vi "生成CODMn data (子VI).vi"() -> (3 "data":T1)   [LabVIEW 2016, in "斯坦道CODMn.lvlib"]
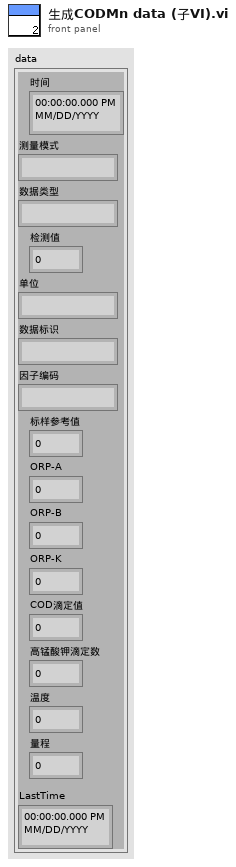
[diagram p1: front panel]
types:
  T1 = cluster{"时间":timestamp, "测量模式":string, "数据类型":string, "检测值":sgl, "单位":string, "数据标识":string, "因子编码":string, "标样参考值":sgl, "ORP-A":sgl, "ORP-B":sgl, "ORP-K":sgl, "COD滴定值":sgl, "高锰酸钾滴定数":sgl, "温度":sgl, "量程":sgl, "LastTime":timestamp}
  T2 = cluster{"运行模式":enum16{"维护模式", "常规模式", "应急模式", "质控模式"}}
  T3 = cluster{"测量量程":dbl, "测量精度":dbl, "测量间隔":dbl, "消解温度":dbl, "消解时长":dbl, "空白校准时间":timestamp, "曲线截距":dbl, "曲线斜率":dbl, "测量检出限":dbl, "测量信号值":dbl, "线性相关系数":dbl, "二次多项式系数":dbl, "标样校准时间":timestamp, "单位":u16}
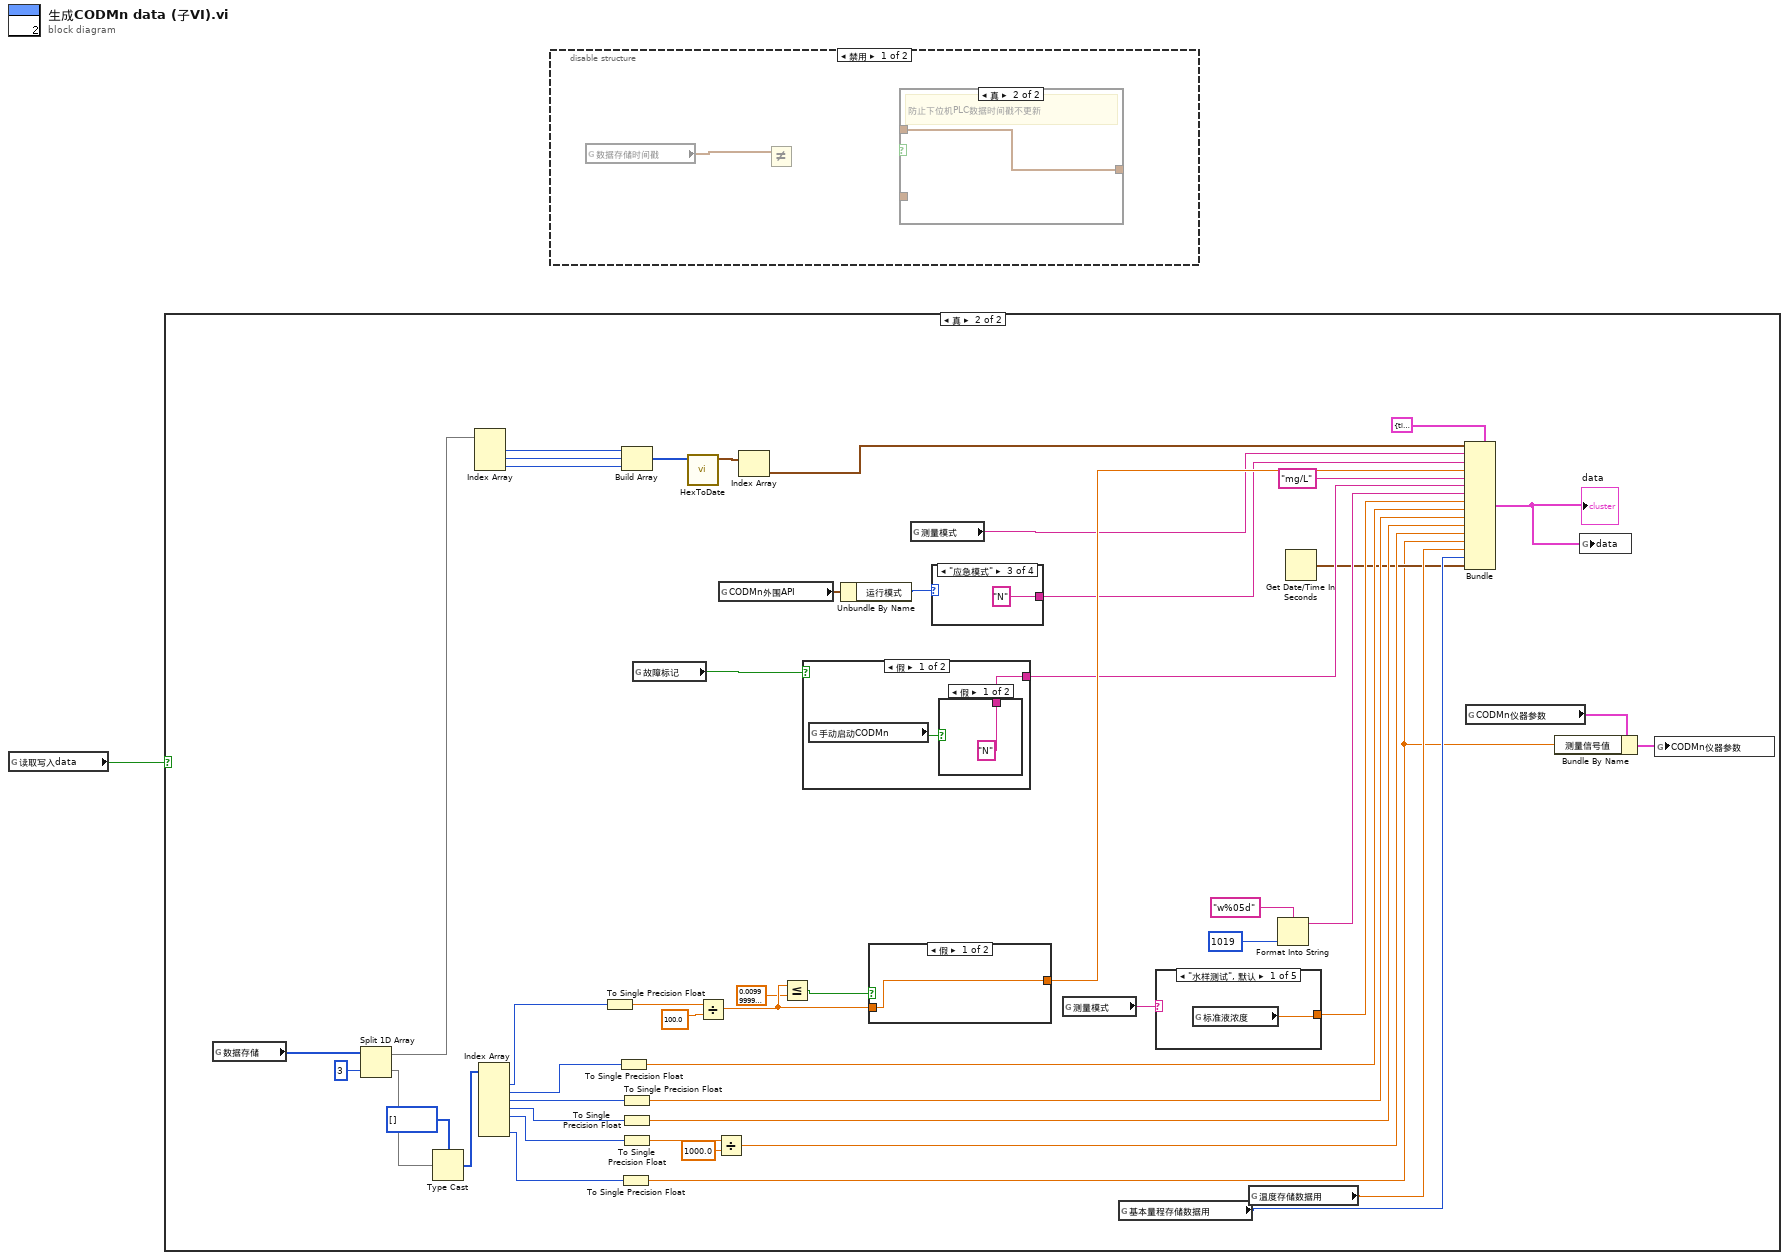
[diagram p0: block diagram]
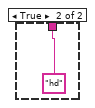
[diagram p5: hidden frame]
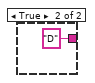
[diagram p6: hidden frame]
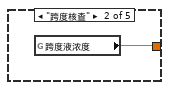
[diagram p7: hidden frame]
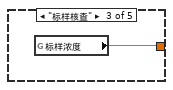
[diagram p8: hidden frame]
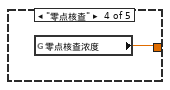
[diagram p9: hidden frame]
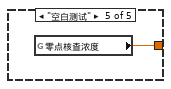
[diagram p10: hidden frame]
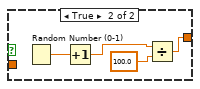
[diagram p11: hidden frame]
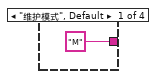
[diagram p12: hidden frame]
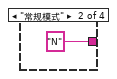
[diagram p13: hidden frame]
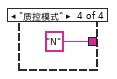
[diagram p14: hidden frame]
diagram:
  n1 = global read "COD内部交互全局.vi" "读取写入data"() -> (w1:bool)
  n2 = case shown="真" w1 {
    frame False {
    }
    frame True {
      n3 = global read "COD内部交互全局.vi" "数据存储"() -> (w9:u16[])
      n4 = Split 1D Array(array=w9, index=3 ("索引")) -> (first subarray=w15:u16[], second subarray=w8:u16[])
      n5 = Type Cast(type=i16[] [], x=w8) -> (*(type *) &x=w7:i16[])
      n6 = Index Array(array=w15) -> (element #1=w17:u16, element #2=w18:u16, element #3=w19:u16)  [unwired: 3 in]
      n7 = Index Array(array=w7) -> (element #1=w42:i16, element #2=w21:i16, element #3=w22:i16, element #4=w23:i16, element #5=w24:i16, element #7=w49:i16)  [unwired: 7 in, 1 out]
      n8 = To Single Precision Float(number=w42) -> (single precision float=w40:sgl)
      n9 = To Single Precision Float(number=w21) -> (single precision float=w33:sgl)
      n10 = To Single Precision Float(number=w49) -> (single precision float=w4:sgl)
      n11 = Build Array(w17, w18, w19) -> (w20:u16[])
      n12 = To Single Precision Float(number=w22) -> (single precision float=w32:sgl)
      n13 = To Single Precision Float(number=w23) -> (single precision float=w31:sgl)
      n14 = To Single Precision Float(number=w24) -> (single precision float=w27:sgl)
      n15 = global read "COD内部交互全局.vi" "故障标记"() -> (w51:bool)
      n16 = call "HexToDate.vi"("数组"=w20) -> ("DATE"=w16:timestamp[])  [unwired: 10 in]
      n17 = Divide(x=w40, y=sgl 100.0) -> (x/y=w41:sgl)
      n18 = Divide(x=w27, y=sgl 1000.0) -> (x/y=w30:sgl)
      n19 = global read "CODMN外部API.vi" "CODMn外围API"() -> (w45:T2)
      n20 = Index Array(array=w16) -> (element=w3:timestamp)  [unwired: 1 in]
      n21 = Less Or Equal?(x=w41, y=sgl 0.01) -> (x <= y?=w39:bool)
      n22 = case shown="假" w51 {
        tunnel: [w53 "D" ("数据标识")] -> w35
        frame False {
          n23 = global read "CODMN外部API.vi" "手动启动CODMn"() -> (w52:bool)
          n24 = case shown="假" w52 {
            tunnel: ["N" ("数据标识") "hd" ("数据标识")] -> w53
            frame False {
            }
            frame True {
            }
          }
        }
        frame True {
        }
      }
      n25 = Unbundle By Name(w45) -> ("运行模式"=w46:enum16{"维护模式", "常规模式", "应急模式", "质控模式"})
      n26 = case shown="假" w39 {
        tunnel: [w62 w63] -> w48
        tunnel: w41 -> [w62 _]
        frame False {
        }
        frame True {
          n27 = Random Number (0-1)() -> (number: 0 to 1=w66:dbl)
          n28 = Increment(x=w66) -> (x+1=w64:dbl)
          n29 = Divide(x=w64, y=sgl 100.0) -> (x/y=w63:dbl)
        }
      }
      n30 = global read "COD测量模式全局.vi" "测量模式"() -> (w47:string)
      n31 = case shown="\"应急模式\"" w46 {
        tunnel: ["M" ("单位") "N" ("单位") "N" ("单位") "N" ("单位")] -> w37
        frame "维护模式", Default {
        }
        frame "常规模式" {
        }
        frame "应急模式" {
        }
        frame "质控模式" {
        }
      }
      n32 = global read "COD测量模式全局.vi" "测量模式"() -> (w43:string)
      n33 = global read "COD内部交互全局.vi" "基本量程存储数据用"() -> (w13:enum16{"L", "H", "AUTO"})
      n34 = case shown="\"水样测试\", 默认" w43 {
        tunnel: [w57 w58 w59 w60 w61] -> w44
        frame "水样测试", Default {
          n35 = global read "COD浓度全局变量.vi" "标准液浓度"() -> (w57:dbl)
        }
        frame "跨度核查" {
          n36 = global read "CODMn断电保存全局变量.vi" "跨度液浓度"() -> (w58:dbl)
        }
        frame "标样核查" {
          n37 = global read "CODMn断电保存全局变量.vi" "标样浓度"() -> (w59:dbl)
        }
        frame "零点核查" {
          n38 = global read "CODMn断电保存全局变量.vi" "零点核查浓度"() -> (w60:dbl)
        }
        frame "空白测试" {
          n39 = global read "CODMn断电保存全局变量.vi" "零点核查浓度"() -> (w61:dbl)
        }
      }
      n40 = global read "COD内部交互全局.vi" "温度存储数据用"() -> (w50:dbl)
      n41 = Format Into String(format string="w%05d" ("格式字符串"), u32 1019 ("因子编码")) -> (resulting string=w34:string)  [unwired: 2 in, 1 out]
      n42 = Get Date/Time In Seconds() -> (seconds since 1Jan1904=w11:timestamp)
      n43 = Bundle(cluster=T1 {"时间"=timestamp(0 s since 1904-01-01), "测量模式"="", "数据类型"="", "检测值"=0.0, "单位"="", "数据标识"="", "因子编码"="", "标样参考值"=0.0, "ORP-A"=0.0, "ORP-B"=0.0, "ORP-K"=0.0, "COD滴定值"=0.0, "高锰酸钾滴定数"=0.0, "温度"=0.0, "量程"=0.0, "LastTime"=timestamp(0 s since 1904-01-01)} ("data"), "时间"=w3, "测量模式"=w47, "数据类型"=w37, "检测值"=w48, "单位"="mg/L", "数据标识"=w35, "因子编码"=w34, "标样参考值"=w44, "ORP-A"=w33, "ORP-B"=w32, "ORP-K"=w31, "COD滴定值"=w30, "高锰酸钾滴定数"=w4, "温度"=w50, "量程"=w13, "LastTime"=w11) -> (w2:T1)
      "data" <- w2
      n44 = global read "CODMn断电保存全局变量.vi" "CODMn仪器参数"() -> (w6:T3)
      n45 = Bundle By Name(cluster=w6, "测量信号值"=w4) -> (w5:T3)
      n46 = global write "COD内部交互全局.vi" "data"(w2) -> ()
      n47 = global write "CODMn断电保存全局变量.vi" "CODMn仪器参数"(w5) -> ()
    }
  }
  n48 = disable-structure shown="禁用" {
    frame Disabled {
      n49 = global read "COD内部交互全局.vi" "数据存储时间戳"() -> (w71:timestamp)
      n50 = Not Equal?(x=w71) -> (x != y?=w72:bool)  [unwired: 1 in]
      n51 = case "条件结构" shown="真" {
        selector: _ -> [_ _]
        tunnel: _ -> [w73 _]
        tunnel: _ -> [_ w74]
        tunnel: [w73 w74] -> _
        frame False {
        }
        frame True {
          # "防止下位机PLC数据时间戳不更新"
        }
      }
    }
    frame Enabled {
    }
  }
